vi "SetFunctionArbs.vi"(8 "error in (no error)":errorcluster, 10 "Variant":variant, 11 "ArbitraryFunction in":refnum<class "ArbitraryFunction.lvclass">) -> (0 "error out":errorcluster, 3 "ArbitraryFunction out":refnum<class "ArbitraryFunction.lvclass">)   [LabVIEW 2018, in "Functions.lvlib" / "ArbitraryFunction.lvclass"]
uses:
  ArbitraryFunction.lvclass
  ArbitraryFunction.lvclass/ArbitraryFunction.ctl
  Accessors/Write SampleRate.vi
  Accessors/Write Arbs.vi
  Accessors/Read Arbs.vi
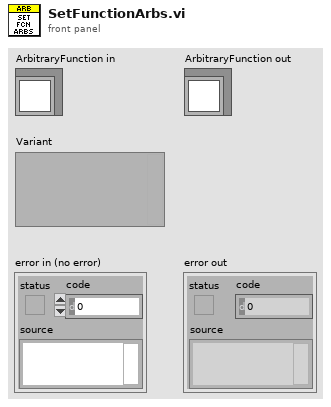
[diagram p1: front panel]
types:
  T1 = cluster{"Arbs":cluster{"Handle":string, "Size":i32, "Gain":dbl, "Offset":dbl}[], "SampleRate":dbl, "SettlingTime":dbl, "T0":dbl}
  T2 = typedef "Functions.lvlib/ArbitraryFunction.lvclass/Arbitrary.ctl" = cluster{"Handle":string, "Size":i32, "Gain":dbl, "Offset":dbl, "Waveform":waveform(dbl)}
  T3 = cluster{"Handle":string, "Size":i32, "Gain":dbl, "Offset":dbl}[]
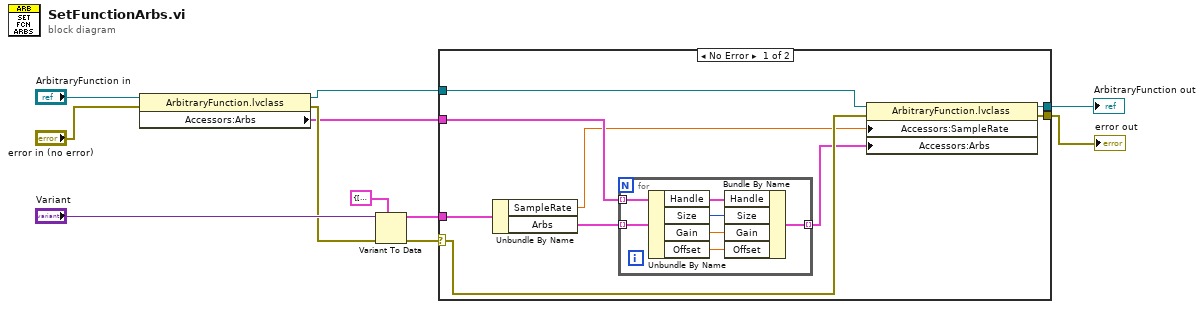
[diagram p0: block diagram]
diagram:
  n1 = property class="ArbitraryFunction.lvclass"(reference="ArbitraryFunction in", error in="error in (no error)") -> (reference out=w5:refnum<class "ArbitraryFunction.lvclass">, error out=w8:errorcluster, "Accessors:Arbs"=w7:T2[])
  n2 = Variant To Data(error in=w8, type=T1 {"Arbs"=[], "SampleRate"=0.0, "SettlingTime"=0.0, "T0"=0.0} ("FunctionConfig"), Variant="Variant") -> (data=w6:T1, error out=w4:errorcluster)
  n3 = case shown="No Error" w4 {
    selector: w4 -> [w17 w28]
    tunnel: w7 -> [w20 _]
    tunnel: w6 -> [w19 _]
    tunnel: w5 -> [w18 w29]
    tunnel: [w16 w28] -> w2
    tunnel: [w15 w29] -> w3
    frame No Error {
      n4 = Unbundle By Name(w19) -> ("SampleRate"=w13:dbl, "Arbs"=w14:T3)
      n5 = for {
        tunnel: w20 -> [w27] mode=indexing
        tunnel: w14 -> [w26] mode=indexing
        tunnel: [w21] -> w12 mode=indexing
        n6 = Unbundle By Name(w26) -> ("Handle"=w25:string, "Size"=w24:i32, "Gain"=w23:dbl, "Offset"=w22:dbl)
        n7 = Bundle By Name(cluster=w27, "Handle"=w25, "Size"=w24, "Gain"=w23, "Offset"=w22) -> (w21:T2)
      }
      n8 = property class="ArbitraryFunction.lvclass"(reference=w18, error in=w17, "Accessors:SampleRate"=w13, "Accessors:Arbs"=w12) -> (reference out=w15:refnum<class "ArbitraryFunction.lvclass">, error out=w16:errorcluster)
    }
    frame Error {
    }
  }
  "error out" <- w2
  "ArbitraryFunction out" <- w3
